vi "Flow cell controller.vi"() -> ()   [LabVIEW 2015]
doc: "User interface to run the Gelles Lab flow cell controller.\n\nModified from original which is Copyright 2005, National Instruments Corporation.\n\nModifications Copyright 2009, Jeff Gelles, Brandeis University"
uses:
  Pump status.ctl
  Current operation.ctl
  Valve position.ctl
  Flow cell controller globals.vi
panel:
  in  "Tab Control":enum32{"Settings", "Operation/Status"}(tab)=enum."Operation/Status"
  in  "Valve # (1=a, etc.)":u8=1
  in  "Pump Address":i32 format="%0#2.0f"
  in  "Pump VISA name":refnum<visa-resource-name>="PUMP"
  in  "Pump Baud Rate":u32(ring)=9600 items=["300"=300, "1200"=1200, "2400"=2400, "9600"=9600]
  in  "Syringe Diameter\n(mm)":dbl=4.61
  in  "Units":u16(ring) items=["microliters per minute (ul/min.)", "microliters per hour (ul/hr.)", "milliliters per minute (ml/min.)", "milliliters per hour (ml/hr.)", "picoliters per minute (pl/min.)", "picoliters per hour (pl/hr.)", "nanoliters per minute (nl/min.)", "nanoliters per hour (nl/hr.)"]
  in  "Syringe Travel\n(mm)":dbl=60.0
  in  "Empty/Wash Syringe Rate":dbl=1200.0
  in  "Valve VISA name":refnum<visa-resource-name>="VALVE"
  in  "Number of valves":i32=1
  in  "Valve Baud Rate":u32(ring)=9600 items=["300"=300, "1200"=1200, "2400"=2400, "9600"=9600]
  in  "Fill syringe with water":bool
  out "Valve position":T1=1 items=["Cell"=1, "Waste"=2, "Water"=3, "Air"=4]
  in  "Start Withdrawing":bool
  in  "Withdraw Rate":dbl=100.0
  out "Flow Rate Units":string
  in  "Fixed volume":bool=TRUE
  in  "Withdraw vol":dbl
  out "Cap units 2":string
  in  "Zero volume readout":bool
  in  "Empty syringe":bool
  out "Syringe position":dbl format="%5.1f"
  out "Units (syr. pos.)":string
  out "Pump model/version":string
  out "Pump status":T2 items=["Error - Can't read status"=-1, "Stopped"=0, "Infusing"=1, "Withdrawing"=2, "Pump stalled"=3, "Stopped at infuse limit"=4, "Stopped at withdraw limit"=5, "Emergency stop"=6, "Stopped at target volume"=7]
  out "Syringe fill %":dbl(slide) scale=0.0..100.0
  out "Syringe capacity":dbl format="%5.1f"
  out "Cap units":string
  out "Current operation":T3
  out "Progress":dbl(slide) scale=0.0..1.0
  out "Valve model/versions":string[](array[string])
  out "Curr op 100%":dbl
  out "Curr op 0%":dbl
  out "Total volume infused since clear":dbl
  out "Total volume withdrawn since clear":dbl
  in  "Quit Program":bool
  in  "Stop Pump":bool
  # "Pump Settings"
  # "Valve Settings"
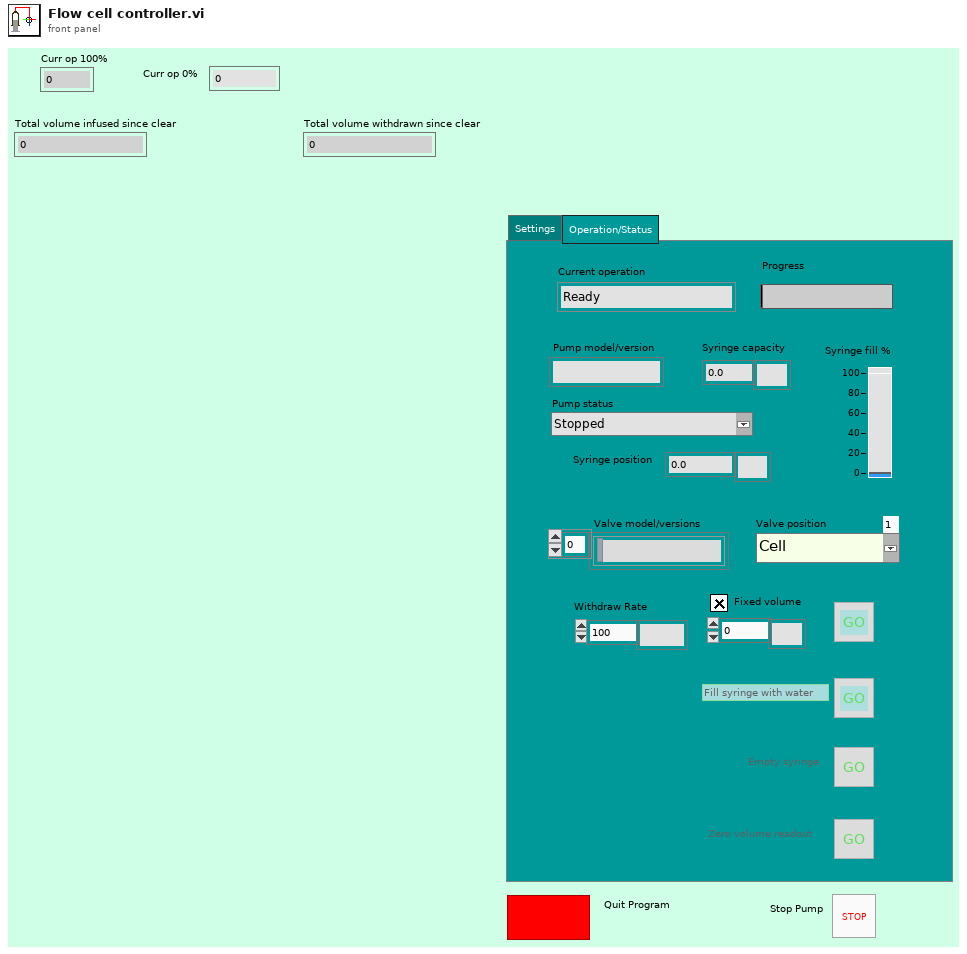
[diagram p1: front panel]
types:
  T1 = typedef "Valve position.ctl" = u16
  T2 = typedef "Pump status.ctl" = i8
  T3 = typedef "Current operation.ctl" = enum16{"Ready", "Flow", "Fixed Volume Flow", "Empty Syringe", "Fill Syringe with Water", "Initializing"}
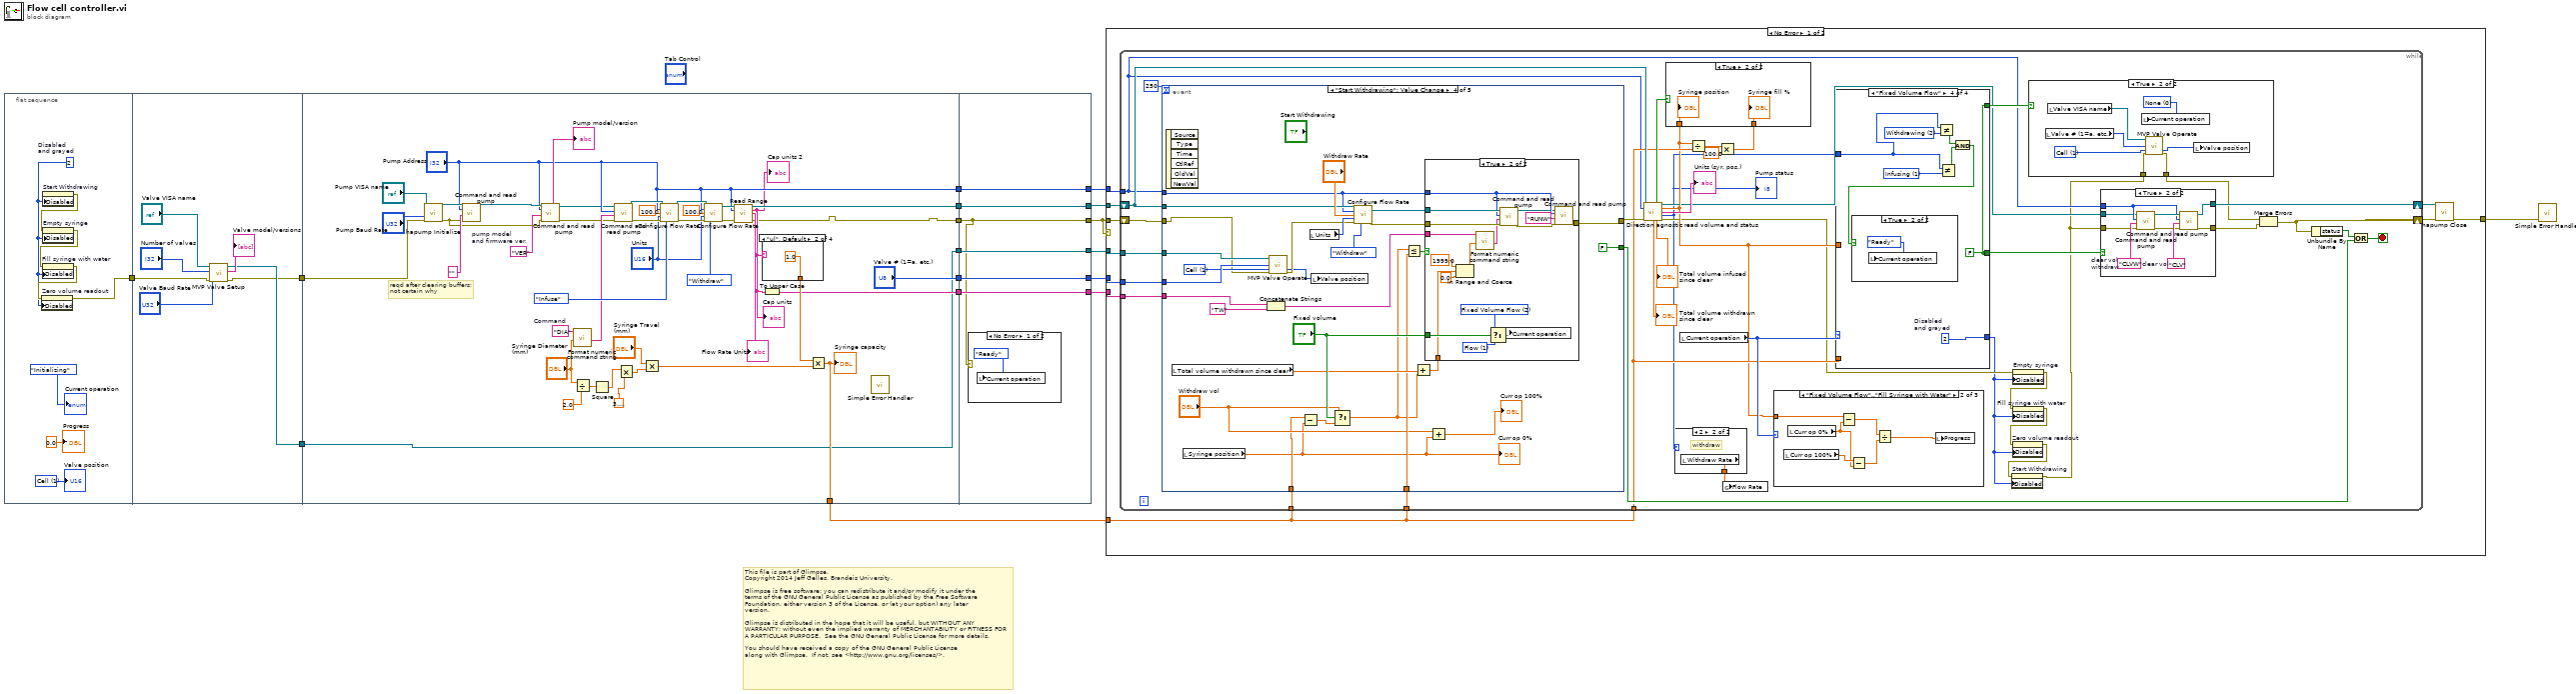
[diagram p0: block diagram]
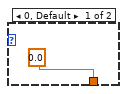
[diagram p2: hidden frame]
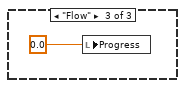
[diagram p6: hidden frame]
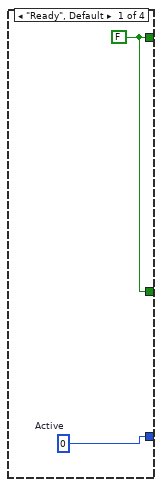
[diagram p7: hidden frame]
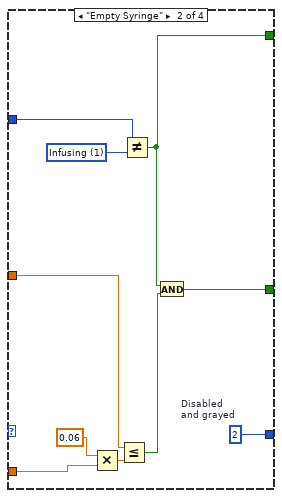
[diagram p8: hidden frame]
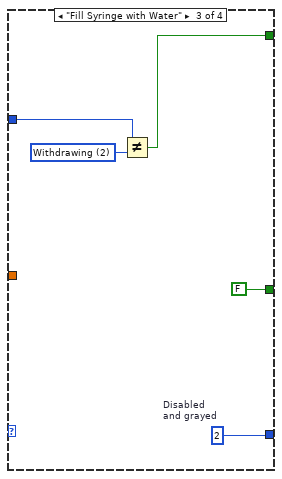
[diagram p9: hidden frame]
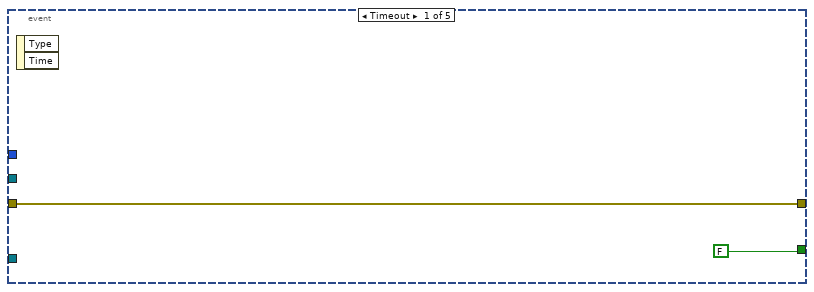
[diagram p12: hidden frame]
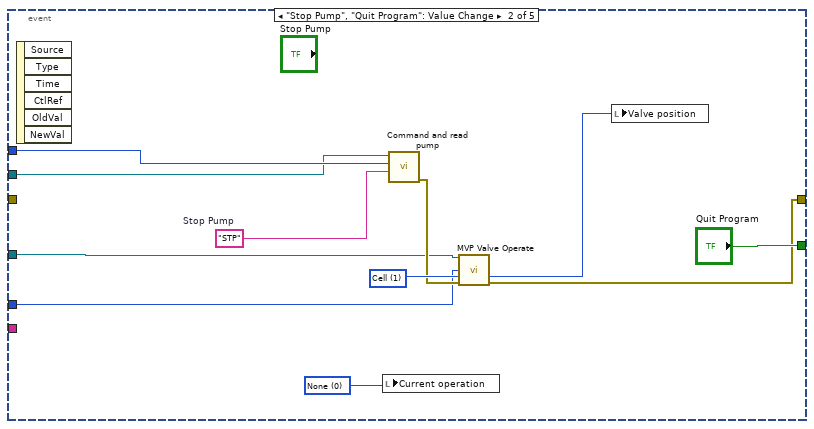
[diagram p13: hidden frame]
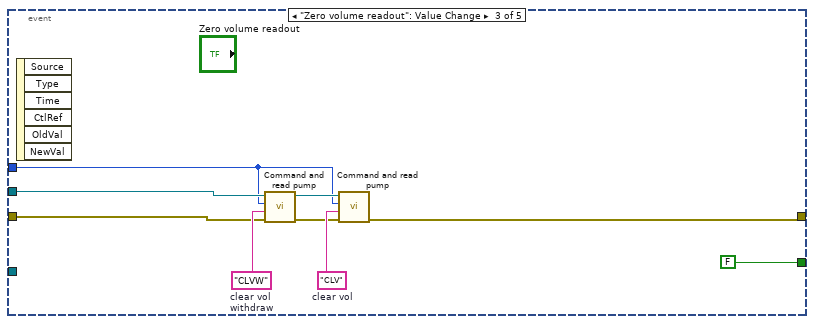
[diagram p14: hidden frame]
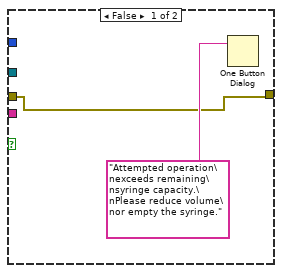
[diagram p15: hidden frame]
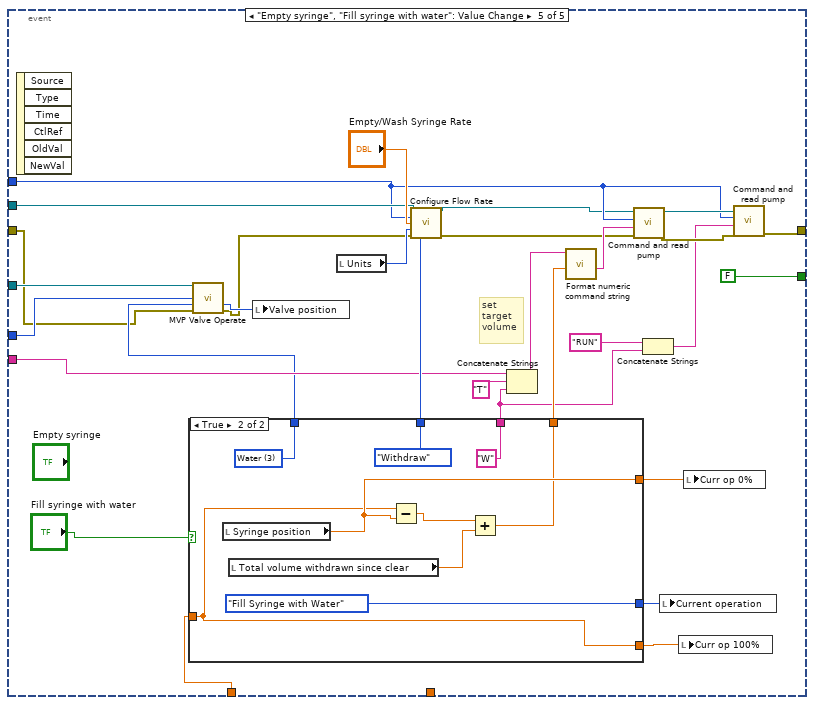
[diagram p16: hidden frame]
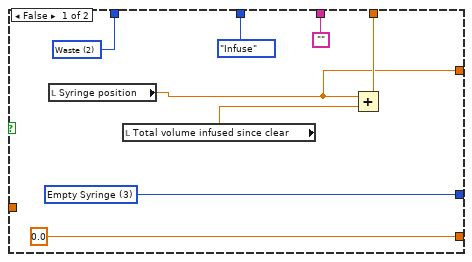
[diagram p17: hidden frame]
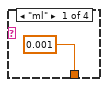
[diagram p19: hidden frame]
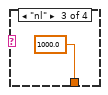
[diagram p20: hidden frame]
diagram:
  # "This file is part of Glimpse. \nCopyright 2014 Jeff Gelles, Brandeis University.    \n\nGlimpse is free software: you can redistribute it and/or modify it under the \nterms of the GNU General Public License as published by the Free Software \nFoundation, either version 3 of the License, or (at your option) any later \nversion.\n\nGlimpse is distributed in the hope that it will be useful, but WITHOUT ANY \nWARRANTY; without even the implied warranty of MERCHANTABILITY or FITNESS FOR \nA PARTICULAR PURPOSE.  See the GNU General Public License for more details.\n\nYou should have received a copy of the GNU General Public License\nalong with Glimpse.  If not, see <http://www.gnu.org/licenses/>."
  n1 = flat-sequence {
    tunnel: [w18] -> w4
    tunnel: w4 -> [w27]
    tunnel: [w26] -> w3
    tunnel: [w28] -> w2
    tunnel: [w40] -> w13
    tunnel: ["Pump Address"] -> w10
    tunnel: [w33] -> w9
    tunnel: [w46] -> w8
    tunnel: [w41] -> w7
    tunnel: [w34] -> w6
    tunnel: ["Valve # (1=a, etc.)"] -> w5
    tunnel: w3 -> [w35]
    tunnel: w2 -> [w34]
    tunnel: [w80] -> w11
    tunnel: [w81] -> w12
    tunnel: [w82] -> w14
    tunnel: [w83] -> w15
    tunnel: [w79] -> w1
    tunnel: [w84] -> w16
    tunnel: w10 -> [w84]
    tunnel: w9 -> [w79]
    tunnel: w8 -> [w83]
    tunnel: w7 -> [w82]
    tunnel: w6 -> [w81]
    tunnel: w5 -> [w80]
    frame #0 {
      w19 = u8 2  # Disabled and grayed
      w23 = u16 1 items=["Cell"=1, "Waste"=2, "Water"=3, "Air"=4] ("Valve position")
      n2 = property on="Start Withdrawing" class="Bool"("Disabled"=w19) -> (error out=w20:errorcluster)  [unwired: 2 in, 1 out]
      n3 = property on="Empty syringe" class="Bool"(error in=w20, "Disabled"=w19) -> (error out=w21:errorcluster)  [unwired: 1 in, 1 out]
      n4 = property on="Fill syringe with water" class="Bool"(error in=w21, "Disabled"=w19) -> (error out=w22:errorcluster)  [unwired: 1 in, 1 out]
      n5 = property on="Zero volume readout" class="Bool"(error in=w22, "Disabled"=w19) -> (error out=w18:errorcluster)  [unwired: 1 in, 1 out]
      "Current operation" <- Current_operation."Initializing" ("Current operation")
      "Progress" <- 0.0 ("Progress")
      "Valve position" <- w23
    }
    frame #1 {
      n6 = call "MVP Valve Setup.vi"("error in (no error)"=w27, "Baud Rate (9600)"="Valve Baud Rate", "Number of valves"="Number of valves", "VISA resource name"="Valve VISA name") -> ("error out"=w26:errorcluster, "Firmware versions"=→"Valve model/versions":string[], "VISA resource name out"=w28:refnum<visa-resource-name>)  [unwired: 5 out]
    }
    frame #2 {
      w60 = "DIA"  # Command
      w62 = "VER"  # pump model and firmware ver.
      # "reqd after clearing buffers; \nnot certain why"
      n7 = call <instrlib>:"hapump Initialize.vi"("VISA resource name"="Pump VISA name", "Baud Rate (9600)"="Pump Baud Rate", "error in (no error)"=w35) -> ("VISA resource name out"=w65:refnum<visa-resource-name>, "error out"=w36:errorcluster)  [unwired: 11 out]
      n8 = call "Command and read pump.vi"("error in (no error)"=w36, "command"="", "Address (00)"="Pump Address", "VISA resource name"=w65) -> ("VISA resource name out"=w64:refnum<visa-resource-name>)  [unwired: 7 out]
      n9 = call "Command and read pump.vi"("error in (no error)"=w36, "command"=w62, "Address (00)"="Pump Address", "VISA resource name"=w64) -> ("error out"=w39:errorcluster, "VISA resource name out"=w38:refnum<visa-resource-name>, "String result"=→"Pump model/version":string)  [unwired: 5 out]
      n10 = call "Format numeric command string.vi"("Number"="Syringe Diameter\n(mm)", "Command"=w60) -> ("String"=w59:string)  [unwired: 5 out]
      n11 = Divide(x="Syringe Diameter\n(mm)", y=2.0) -> (x/y=w55:dbl)
      n12 = Square(x=w55) -> (x^2=w54:dbl)
      n13 = call "Command and read pump.vi"("error in (no error)"=w39, "command"=w59, "Address (00)"="Pump Address", "VISA resource name"=w38) -> ("error out"=w72:errorcluster, "VISA resource name out"=w73:refnum<visa-resource-name>)  [unwired: 6 out]
      n14 = Multiply(x=w54, y=3.141592653589793) -> (x*y=w53:dbl)
      n15 = Multiply(x="Syringe Travel\n(mm)", y=w53) -> (x*y=w44:dbl)
      n16 = call "Configure Flow Rate.vi"("VISA resource name"=w73, "Address (00)"="Pump Address", "Flow Rate (100)"=100.0, "Units (0: microliters per minute)"="Units", "error in (no error)"=w72, "Pump direction"=enum16{"Infuse", "Withdraw"}."Infuse") -> ("VISA resource name out"=w69:refnum<visa-resource-name>, "error out"=w68:errorcluster)  [unwired: 8 out]
      n17 = call "Configure Flow Rate.vi"("VISA resource name"=w69, "Address (00)"="Pump Address", "Flow Rate (100)"=100.0, "Units (0: microliters per minute)"="Units", "error in (no error)"=w68, "Pump direction"=enum16{"Infuse", "Withdraw"}."Withdraw") -> ("VISA resource name out"=w49:refnum<visa-resource-name>, "error out"=w47:errorcluster)  [unwired: 8 out]
      n18 = call "Read Range.vi"("VISA resource name"=w49, "Address (00)"="Pump Address", "error in (no error)"=w47) -> ("VISA resource name out"=w46:refnum<visa-resource-name>, "Target Units"=w42:string, "Flow Rate Units"=→"Flow Rate Units":string, "error out"=w33:errorcluster)  [unwired: 9 out]
      "Cap units" <- w42
      "Cap units 2" <- w42
      n19 = case shown="\"ul\", Default" w42 {
        tunnel: [0.001 ("y") 1.0 ("y") 1000.0 ("y") 1000000.0 ("y")] -> w45
        frame "ml" {
        }
        frame "ul", Default {
        }
        frame "nl" {
        }
        frame "pl" {
        }
      }
      n20 = To Upper Case(1:w42) -> (0:w41:string)
      n21 = Multiply(x=w45, y=w44) -> (x*y=w40:dbl)
      "Syringe capacity" <- w40
      n22 = call <vilib>:"Simple Error Handler.vi"() -> ()  [unwired: 5 in, 5 out]
    }
    frame #3 {
      n23 = case shown="No Error" w79 {
        frame No Error {
          n24 = local write "Current operation"(Current_operation."Ready" ("Current operation")) -> ()
        }
        frame Error {
        }
      }
    }
  }
  n25 = case shown="No Error" w1 {
    tunnel: [w95 w307] -> w17
    tunnel: w16 -> [w92 _]
    tunnel: w1 -> [w91 w307]
    tunnel: w15 -> [w90 _]
    tunnel: w14 -> [w89 _]
    tunnel: w13 -> [w88 _]
    tunnel: w12 -> [w87 _]
    tunnel: w11 -> [w86 _]
    frame No Error {
      n26 = while {
        tunnel: w92 -> [w111]
        shift-right: [w108] -> w93
        shift-left: w91 -> [w133]
        shift-right: [w110] -> w94
        shift-left: w90 -> [w126]
        tunnel: w88 -> [w117]
        tunnel: w89 -> [w124]
        tunnel: w88 -> [w123]
        tunnel: w88 -> [w118]
        tunnel: w87 -> [w114]
        tunnel: w86 -> [w115]
        stop <- w129 stop-if-true
        n27 = event shown="[3] \"Start Withdrawing\": Value Change" {
          selector: _ -> [_ _ _ _ _]
          dyn-events: _ -> [_ _ _ _ _]
          timeout: 250 -> [_ _ _ _ _]
          tunnel: w111 -> [_ w201 w205 w233 w276]
          tunnel: w126 -> [_ w200 w209 w235 w285]
          tunnel: w133 -> [w190 _ w210 w220 w267]
          tunnel: [w190 w195 w203 w239 w288] -> w127
          tunnel: [FALSE "Quit Program" FALSE ("Quit Program") FALSE ("Quit Program") FALSE ("Quit Program")] -> w130
          tunnel: w124 -> [_ _ _ w230 w283]
          tunnel: w123 -> [_ _ _ w213 w260]
          tunnel: w118 -> [_ _ _ w224 _]
          tunnel: w115 -> [_ w193 _ w223 w268]
          tunnel: w114 -> [_ w194 _ w222 w269]
          event Timeout {
            n28 = event-data() -> ()  [unwired: 3 out]
          }
          event "Stop Pump", "Quit Program": Value Change {
            w197 = u16 1 items=["Cell"=1, "Waste"=2, "Water"=3, "Air"=4] ("Valve position")
            w198 = u16 0 items=["None", "Flow", "Fixed Volume Flow", "Empty Syringe"] ("Current operation")
            w199 = "STP"  # Stop Pump
            n29 = event-data() -> ()  [unwired: 7 out]
            n30 = local write "Current operation"(w198) -> ()
            n31 = call "Command and read pump.vi"("command"=w199, "Address (00)"=w201, "VISA resource name"=w200) -> ("error out"=w196:errorcluster)  [unwired: 1 in, 7 out]
            n32 = call "MVP Valve Operate.vi"("VISA resource name"=w194, "Valve # (1=a, 2=b, ....  0 = no prefix)"=w193, "Valve position in"=w197, "error in (no error)"=w196) -> ("Valve position out"=w192:u8, "error out"=w195:errorcluster)  [unwired: 10 out]
            n33 = local write "Valve position"(w192) -> ()
          }
          event "Zero volume readout": Value Change {
            w207 = "CLV"  # clear vol
            w211 = "CLVW"  # clear vol withdraw
            n34 = event-data() -> ()  [unwired: 7 out]
            n35 = call "Command and read pump.vi"("error in (no error)"=w210, "command"=w211, "Address (00)"=w205, "VISA resource name"=w209) -> ("error out"=w204:errorcluster, "VISA resource name out"=w206:refnum<visa-resource-name>)  [unwired: 6 out]
            n36 = call "Command and read pump.vi"("error in (no error)"=w204, "command"=w207, "Address (00)"=w205, "VISA resource name"=w206) -> ("error out"=w203:errorcluster)  [unwired: 7 out]
          }
          event "Start Withdrawing": Value Change {
            w221 = u16 1 items=["Cell"=1, "Waste"=2, "Water"=3, "Air"=4] ("Valve position")
            n37 = event-data() -> ()  [unwired: 7 out]
            n38 = local read "Total volume withdrawn since clear"() -> (w225:dbl)
            n39 = local read "Syringe position"() -> (w212:dbl)
            "Curr op 0%" <- w212
            n40 = Concatenate Strings(w230, "TW" ("Command")) -> (w229:string)
            n41 = call "MVP Valve Operate.vi"("VISA resource name"=w222, "Valve # (1=a, 2=b, ....  0 = no prefix)"=w223, "Valve position in"=w221, "error in (no error)"=w220) -> ("Valve position out"=w218:u8, "error out"=w219:errorcluster)  [unwired: 10 out]
            n42 = Subtract(x=w213, y=w212) -> (x-y=w214:dbl)
            n43 = local read "Units"() -> (w237:u16)
            n44 = local write "Valve position"(w218) -> ()
            n45 = Select(t="Withdraw vol", s="Fixed volume", f=w214) -> (s? t:f=w217:dbl)
            n46 = call "Configure Flow Rate.vi"("VISA resource name"=w235, "Address (00)"=w233, "Flow Rate (100)"="Withdraw Rate", "Units (0: microliters per minute)"=w237, "error in (no error)"=w219, "Pump direction"=enum16{"Infuse", "Withdraw"}."Withdraw") -> ("VISA resource name out"=w234:refnum<visa-resource-name>, "error out"=w232:errorcluster)  [unwired: 8 out]
            n47 = Less Or Equal?(x=w217, y=w224) -> (x <= y?=w228:bool)
            n48 = Add(x=w225, y=w217) -> (x+y=w216:dbl)
            n49 = case shown="True" w228 {
              tunnel: [w241 w258] -> w239
              tunnel: w234 -> [_ w257]
              tunnel: w233 -> [_ w256]
              tunnel: w232 -> [w241 w255]
              tunnel: w229 -> [_ w252]
              tunnel: w216 -> [_ w244]
              tunnel: "Fixed volume" -> [_ w250]
              frame False {
                n50 = One Button Dialog(message="Attempted operation\nexceeds remaining\nsyringe capacity.\nPlease reduce volume\nor empty the syringe.") -> ()  [unwired: 2 out]
              }
              frame True {
                w249 = u16 1 items=["None", "Flow", "Fixed Volume Flow", "Empty Syringe"] ("Current operation")
                w248 = u16 2 items=["None", "Flow", "Fixed Volume Flow", "Empty Syringe"] ("Current operation")
                n51 = In Range and Coerce(upper limit=1999.0, x=w244, lower limit=0.0) -> (coerced(x)=w243:dbl)  [unwired: 1 out]
                n52 = call "Format numeric command string.vi"("Number"=w243, "Command"=w252) -> ("String"=w251:string)  [unwired: 5 out]
                n53 = Select(t=w248, s=w250, f=w249) -> (s? t:f=w247:u16)
                n54 = call "Command and read pump.vi"("error in (no error)"=w255, "command"=w251, "Address (00)"=w256, "VISA resource name"=w257) -> ("error out"=w253:errorcluster, "VISA resource name out"=w254:refnum<visa-resource-name>)  [unwired: 6 out]
                n55 = local write "Current operation"(w247) -> ()
                n56 = call "Command and read pump.vi"("error in (no error)"=w253, "command"="RUNW", "Address (00)"=w256, "VISA resource name"=w254) -> ("error out"=w258:errorcluster)  [unwired: 7 out]
              }
            }
            n57 = Add(x="Withdraw vol", y=w212) -> (x+y=→"Curr op 100%":dbl)
          }
          event "Empty syringe", "Fill syringe with water": Value Change {
            # "set\ntarget\nvolume"
            n58 = event-data() -> ()  [unwired: 7 out]
            n59 = case shown="True" "Fill syringe with water" {
              tunnel: [enum16{"Infuse", "Withdraw"}."Infuse" ("Pump direction") enum16{"Infuse", "Withdraw"}."Withdraw" ("Pump direction")] -> w287
              tunnel: [w296 Current_operation."Fill Syringe with Water" ("Current operation")] -> w277
              tunnel: [w295 w300] -> w273
              tunnel: [w293 w302] -> w272
              tunnel: [0.0 ("Curr op 100%") w299] -> w271
              tunnel: [w291 w305] -> w270
              tunnel: ["" "W" ("string")] -> w261
              tunnel: w260 -> [_ w299]
              frame False {
                w291 = u16 2 items=["Cell"=1, "Waste"=2, "Water"=3, "Air"=4] ("Valve position")
                w296 = u16 3 items=["None", "Flow", "Fixed Volume Flow", "Empty Syringe"] ("Current operation")
                n60 = local read "Syringe position"() -> (w293:dbl)
                n61 = local read "Total volume infused since clear"() -> (w294:dbl)
                n62 = Add(x=w293, y=w294) -> (x+y=w295:dbl)
              }
              frame True {
                w305 = u16 3 items=["Cell"=1, "Waste"=2, "Water"=3, "Air"=4] ("Valve position")
                n63 = local read "Syringe position"() -> (w302:dbl)
                n64 = local read "Total volume withdrawn since clear"() -> (w304:dbl)
                n65 = Subtract(x=w299, y=w302) -> (x-y=w301:dbl)
                n66 = Add(x=w301, y=w304) -> (x+y=w300:dbl)
              }
            }
            n67 = call "MVP Valve Operate.vi"("VISA resource name"=w269, "Valve # (1=a, 2=b, ....  0 = no prefix)"=w268, "Valve position in"=w270, "error in (no error)"=w267) -> ("Valve position out"=w265:u8, "error out"=w264:errorcluster)  [unwired: 10 out]
            n68 = local write "Valve position"(w265) -> ()
            n69 = local read "Units"() -> (w266:u16)
            n70 = call "Configure Flow Rate.vi"("VISA resource name"=w285, "Address (00)"=w276, "Flow Rate (100)"="Empty/Wash Syringe Rate", "Units (0: microliters per minute)"=w266, "error in (no error)"=w264, "Pump direction"=w287) -> ("VISA resource name out"=w274:refnum<visa-resource-name>, "error out"=w275:errorcluster)  [unwired: 8 out]
            n71 = Concatenate Strings(w283, "T" ("Command"), w261) -> (w282:string)
            n72 = call "Format numeric command string.vi"("Number"=w273, "Command"=w282) -> ("String"=w278:string)  [unwired: 5 out]
            n73 = call "Command and read pump.vi"("error in (no error)"=w275, "command"=w278, "Address (00)"=w276, "VISA resource name"=w274) -> ("error out"=w279:errorcluster, "VISA resource name out"=w280:refnum<visa-resource-name>)  [unwired: 6 out]
            n74 = Concatenate Strings("RUN" ("command"), w261) -> (w262:string)
            n75 = local write "Current operation"(w277) -> ()
            n76 = local write "Curr op 100%"(w271) -> ()
            n77 = local write "Curr op 0%"(w272) -> ()
            n78 = call "Command and read pump.vi"("error in (no error)"=w279, "command"=w262, "Address (00)"=w276, "VISA resource name"=w280) -> ("error out"=w288:errorcluster)  [unwired: 7 out]
          }
        }
        n79 = call "Direction agnostic read volume and status.vi"("VISA resource name"=w126, "Address (00)"=w111, "error in (no error)"=w127) -> ("Vol OK?"=w122:bool, "VISA resource name out"=w106:refnum<visa-resource-name>, "Volume"=w116:dbl, "Units"=→"Units (syr. pos.)":string, "Pump status"=w97:T2, "Total volume withdrawn since clear"=→"Total volume withdrawn since clear":dbl, "Total volume infused since clear"=→"Total volume infused since clear":dbl, "error out"=w100:errorcluster)  [unwired: 1 in, 4 out]
        "Pump status" <- w97
        n80 = case shown="2" w97 {
          tunnel: [0.0 ("Flow Rate") w135] -> w96
          frame 0, Default {
          }
          frame 2 {
            # "withdraw"
            n81 = local read "Withdraw Rate"() -> (w135:dbl)
          }
        }
        n82 = local read "Current operation"() -> (w119:T3)
        n83 = Divide(x=w116, y=w117) -> (x/y=w125:dbl)
        n84 = Multiply(x=w125, y=100.0) -> (x*y=w105:dbl)
        n85 = case shown="True" w122 {
          tunnel: w105 -> [_ w189]
          tunnel: w116 -> [_ w188]
          frame False {
          }
          frame True {
            "Syringe position" <- w188
            "Syringe fill %" <- w189
          }
        }
        n86 = global write "Flow cell controller globals.vi" "Flow Rate"(w96) -> ()
        n87 = case shown="\"Fixed Volume Flow\"..\"Fill Syringe with Water\"" w119 {
          tunnel: w116 -> [_ w160 _]
          frame "Ready", Default {
          }
          frame "Fixed Volume Flow".."Fill Syringe with Water" {
            n88 = local read "Curr op 100%"() -> (w159:dbl)
            n89 = local read "Curr op 0%"() -> (w158:dbl)
            n90 = Subtract(x=w160, y=w158) -> (x-y=w156:dbl)
            n91 = Subtract(x=w159, y=w158) -> (x-y=w157:dbl)
            n92 = Divide(x=w156, y=w157) -> (x/y=w155:dbl)
            n93 = local write "Progress"(w155) -> ()
          }
          frame "Flow" {
            n94 = local write "Progress"(0.0 ("Progress")) -> ()
          }
        }
        n95 = case shown="\"Fixed Volume Flow\"" w119 {
          tunnel: w97 -> [_ w172 w177 w184]
          tunnel: w117 -> [_ w171 _ _]
          tunnel: w116 -> [_ w168 _ _]
          tunnel: [w163 w166 FALSE w180] -> w113
          tunnel: [w163 w165 w176 w180] -> w112
          tunnel: [w162 w164 w174 w179] -> w98
          frame "Ready", Default {
            w162 = u8 0  # Active
            w163 = FALSE
          }
          frame "Empty Syringe" {
            w164 = u8 2  # Disabled and grayed
            w173 = T2 1 items=["Error - Can't read status"=-1, "Stopped"=0, "Infusing"=1, "Withdrawing"=2, "Pump stalled"=3, "Stopped at infuse limit"=4, "Stopped at withdraw limit"=5, "Emergency stop"=6, "Stopped at target volume"=7] ("y")
            n96 = Multiply(x=0.06, y=w171) -> (x*y=w169:dbl)
            n97 = Less Or Equal?(x=w168, y=w169) -> (x <= y?=w167:bool)
            n98 = Not Equal?(x=w172, y=w173) -> (x != y?=w165:bool)
            n99 = And(x=w165, y=w167) -> (x .and. y?=w166:bool)
          }
          frame "Fill Syringe with Water" {
            w174 = u8 2  # Disabled and grayed
            w178 = T2 2 items=["Error - Can't read status"=-1, "Stopped"=0, "Infusing"=1, "Withdrawing"=2, "Pump stalled"=3, "Stopped at infuse limit"=4, "Stopped at withdraw limit"=5, "Emergency stop"=6, "Stopped at target volume"=7] ("y")
            n100 = Not Equal?(x=w177, y=w178) -> (x != y?=w176:bool)
          }
          frame "Fixed Volume Flow" {
            w179 = u8 2  # Disabled and grayed
            w180 = FALSE
            w185 = T2 2 items=["Error - Can't read status"=-1, "Stopped"=0, "Infusing"=1, "Withdrawing"=2, "Pump stalled"=3, "Stopped at infuse limit"=4, "Stopped at withdraw limit"=5, "Emergency stop"=6, "Stopped at target volume"=7] ("y")
            w186 = T2 1 items=["Error - Can't read status"=-1, "Stopped"=0, "Infusing"=1, "Withdrawing"=2, "Pump stalled"=3, "Stopped at infuse limit"=4, "Stopped at withdraw limit"=5, "Emergency stop"=6, "Stopped at target volume"=7] ("y")
            n101 = Not Equal?(x=w184, y=w185) -> (x != y?=w182:bool)
            n102 = Not Equal?(x=w184, y=w186) -> (x != y?=w181:bool)
            n103 = And(x=w182, y=w181) -> (x .and. y?=w183:bool)
            n104 = case shown="True" w183 {
              frame False {
              }
              frame True {
                n105 = local write "Current operation"(Current_operation."Ready" ("Current operation")) -> ()
              }
            }
          }
        }
        n106 = property on="Empty syringe" class="Bool"(error in=w100, "Disabled"=w98) -> (error out=w101:errorcluster)  [unwired: 1 in, 1 out]
        n107 = property on="Fill syringe with water" class="Bool"(error in=w101, "Disabled"=w98) -> (error out=w102:errorcluster)  [unwired: 1 in, 1 out]
        n108 = property on="Zero volume readout" class="Bool"(error in=w102, "Disabled"=w98) -> (error out=w103:errorcluster)  [unwired: 1 in, 1 out]
        n109 = property on="Start Withdrawing" class="Bool"(error in=w103, "Disabled"=w98) -> (error out=w99:errorcluster)  [unwired: 1 in, 1 out]
        n110 = case shown="True" w112 {
          tunnel: w99 -> [w136 w142]
          tunnel: [w136 w141] -> w107
          frame False {
          }
          frame True {
            w140 = u16 1 items=["Cell"=1, "Waste"=2, "Water"=3, "Air"=4] ("Valve position")
            w143 = u16 0 items=["None", "Flow", "Fixed Volume Flow", "Empty Syringe"] ("Current operation")
            n111 = local read "Valve # (1=a, etc.)"() -> (w139:u8)
            n112 = local read "Valve VISA name"() -> (w138:refnum<visa-resource-name>)
            n113 = local write "Current operation"(w143) -> ()
            n114 = call "MVP Valve Operate.vi"("VISA resource name"=w138, "Valve # (1=a, 2=b, ....  0 = no prefix)"=w139, "Valve position in"=w140, "error in (no error)"=w142) -> ("Valve position out"=w137:u8, "error out"=w141:errorcluster)  [unwired: 10 out]
            n115 = local write "Valve position"(w137) -> ()
          }
        }
        n116 = case shown="True" w113 {
          tunnel: w99 -> [w145 w150]
          tunnel: w111 -> [_ w149]
          tunnel: [w145 w148] -> w109
          tunnel: [w144 w147] -> w110
          tunnel: w106 -> [w144 w146]
          frame False {
          }
          frame True {
            w153 = "CLV"  # clear vol
            w154 = "CLVW"  # clear vol withdraw
            n117 = call "Command and read pump.vi"("error in (no error)"=w150, "command"=w154, "Address (00)"=w149, "VISA resource name"=w146) -> ("error out"=w151:errorcluster, "VISA resource name out"=w152:refnum<visa-resource-name>)  [unwired: 6 out]
            n118 = call "Command and read pump.vi"("error in (no error)"=w151, "command"=w153, "Address (00)"=w149, "VISA resource name"=w152) -> ("error out"=w148:errorcluster, "VISA resource name out"=w147:refnum<visa-resource-name>)  [unwired: 6 out]
          }
        }
        n119 = Merge Errors(w107, w109) -> (w108:errorcluster)
        n120 = Unbundle By Name(w108) -> ("status"=w131:bool)
        n121 = Or(x=w131, y=w130) -> (x .or. y?=w129:bool)
      }
      n122 = call <instrlib>:"hapump Close.vi"("VISA resource name"=w94, "error in (no error)"=w93) -> ("error out"=w95:errorcluster)  [unwired: 13 out]
    }
    frame Error {
    }
  }
  n123 = call <vilib>:"Simple Error Handler.vi"("error in (no error)"=w17) -> ()  [unwired: 1 in, 8 out]
